vi "status_msg.vi"(11 "status_Word":u16) -> (3 "controlMsg":string)   [LabVIEW 2023, in "pump_Lib.lvlib"]
uses:
  pump_Lib.lvlib
panel:
  in  "errors_List":string[][](array[string])=[["0", " "], ["100", "Нет связи!"], ["101", "Стоп объём"], ["102", "Стоп ШВП"], ["103", "Стоп Pmax"], ["104", "Домой"], ["105", "Ошибка привода"], ["106", "Ошибка привода"], ["107", "Ошибка АЦП"], ["108", "Фильтрация"], ["109", "Откачка"], ["110", "Подготовка"], ["111", "Работа"], ["210", "Ожидание"]]
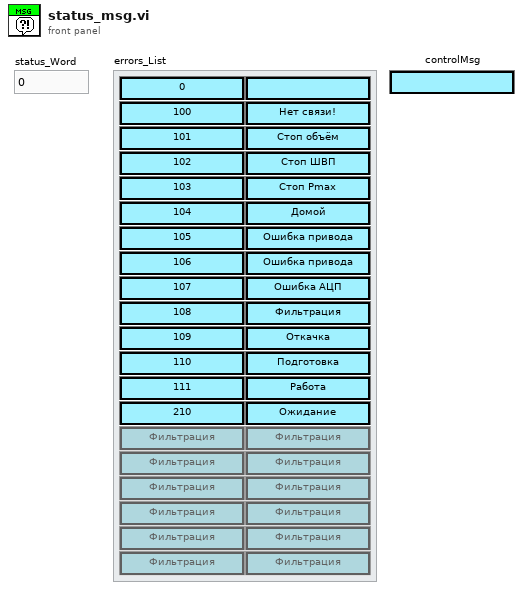
[diagram p1: front panel]
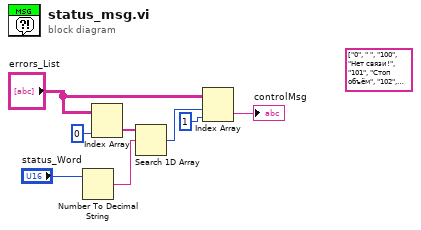
[diagram p0: block diagram]
diagram:
  (unwired) string[][] [["0", " "], ["100", "Нет связи!"], ["101", "Стоп объём"], ["102", "Стоп ШВП"], ["103", "Стоп Pmax"], ["104", "Домой"], ["105", "Ошибка привода"], ["106", "Ошибка привода"], ["107", "Ошибка АЦП"], ["108", "Фильтрация"], ["109", "Откачка"], ["110", "Подготовка"], ["111", "Работа"], ["210", "Ожидание"]] ("errors_List")
  n1 = Number To Decimal String(number="status_Word") -> (decimal integer string=w7:string)  [unwired: 1 in]
  n2 = Index Array(array="errors_List", index (col)=0 ("index (row)")) -> (element=w8:string[])  [unwired: 1 in]
  n3 = Search 1D Array(1D array=w8, element=w7) -> (index of element=w4:i32)  [unwired: 1 in]
  n4 = Index Array(array="errors_List", index (row)=w4, index (col)=1 ("disabled index (row)")) -> (element=→"controlMsg":string)
